vi "获取MPPT状态.vi"(8 "error in (no error)":errorcluster, 11 "MB session in":refnum<class "MB_Master.lvclass">) -> (0 "error out":errorcluster, 1 "结果字符串":string caption="状态", 2 "状态":T1, 3 "MB session out":refnum<class "MB_Master.lvclass">)   [LabVIEW 2016, in "采配水.lvlib"]
uses:
  <vilib>/Plasmionique/MB Master/MB_Master/MB_Master.lvclass
  <vilib>/Plasmionique/MB Master/MB Master.lvlib
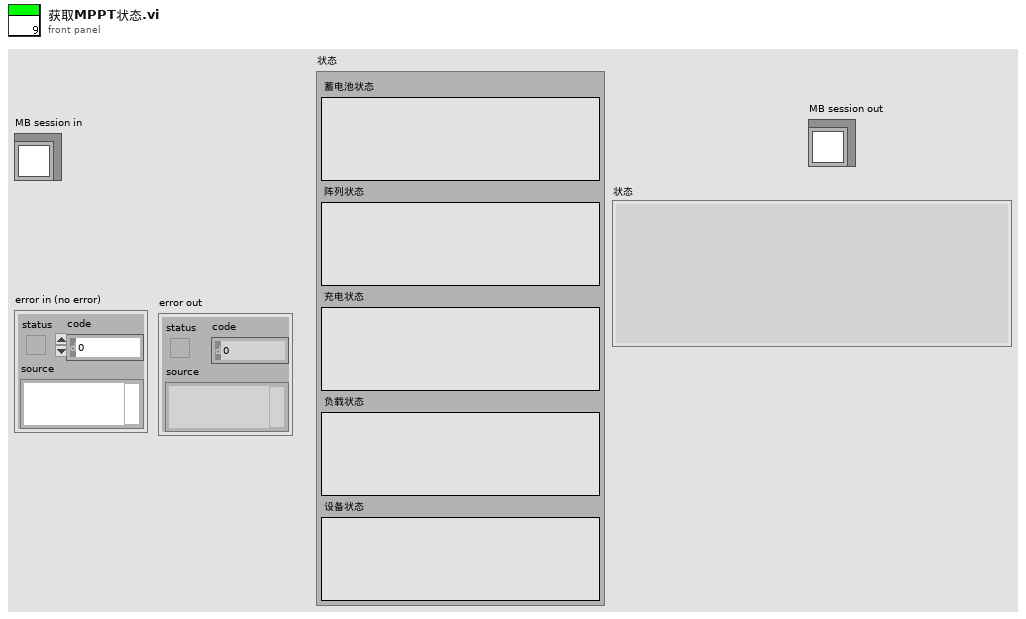
[diagram p1: front panel]
types:
  T1 = cluster{"蓄电池状态":string, "阵列状态":string, "充电状态":string, "负载状态":string, "设备状态":string}
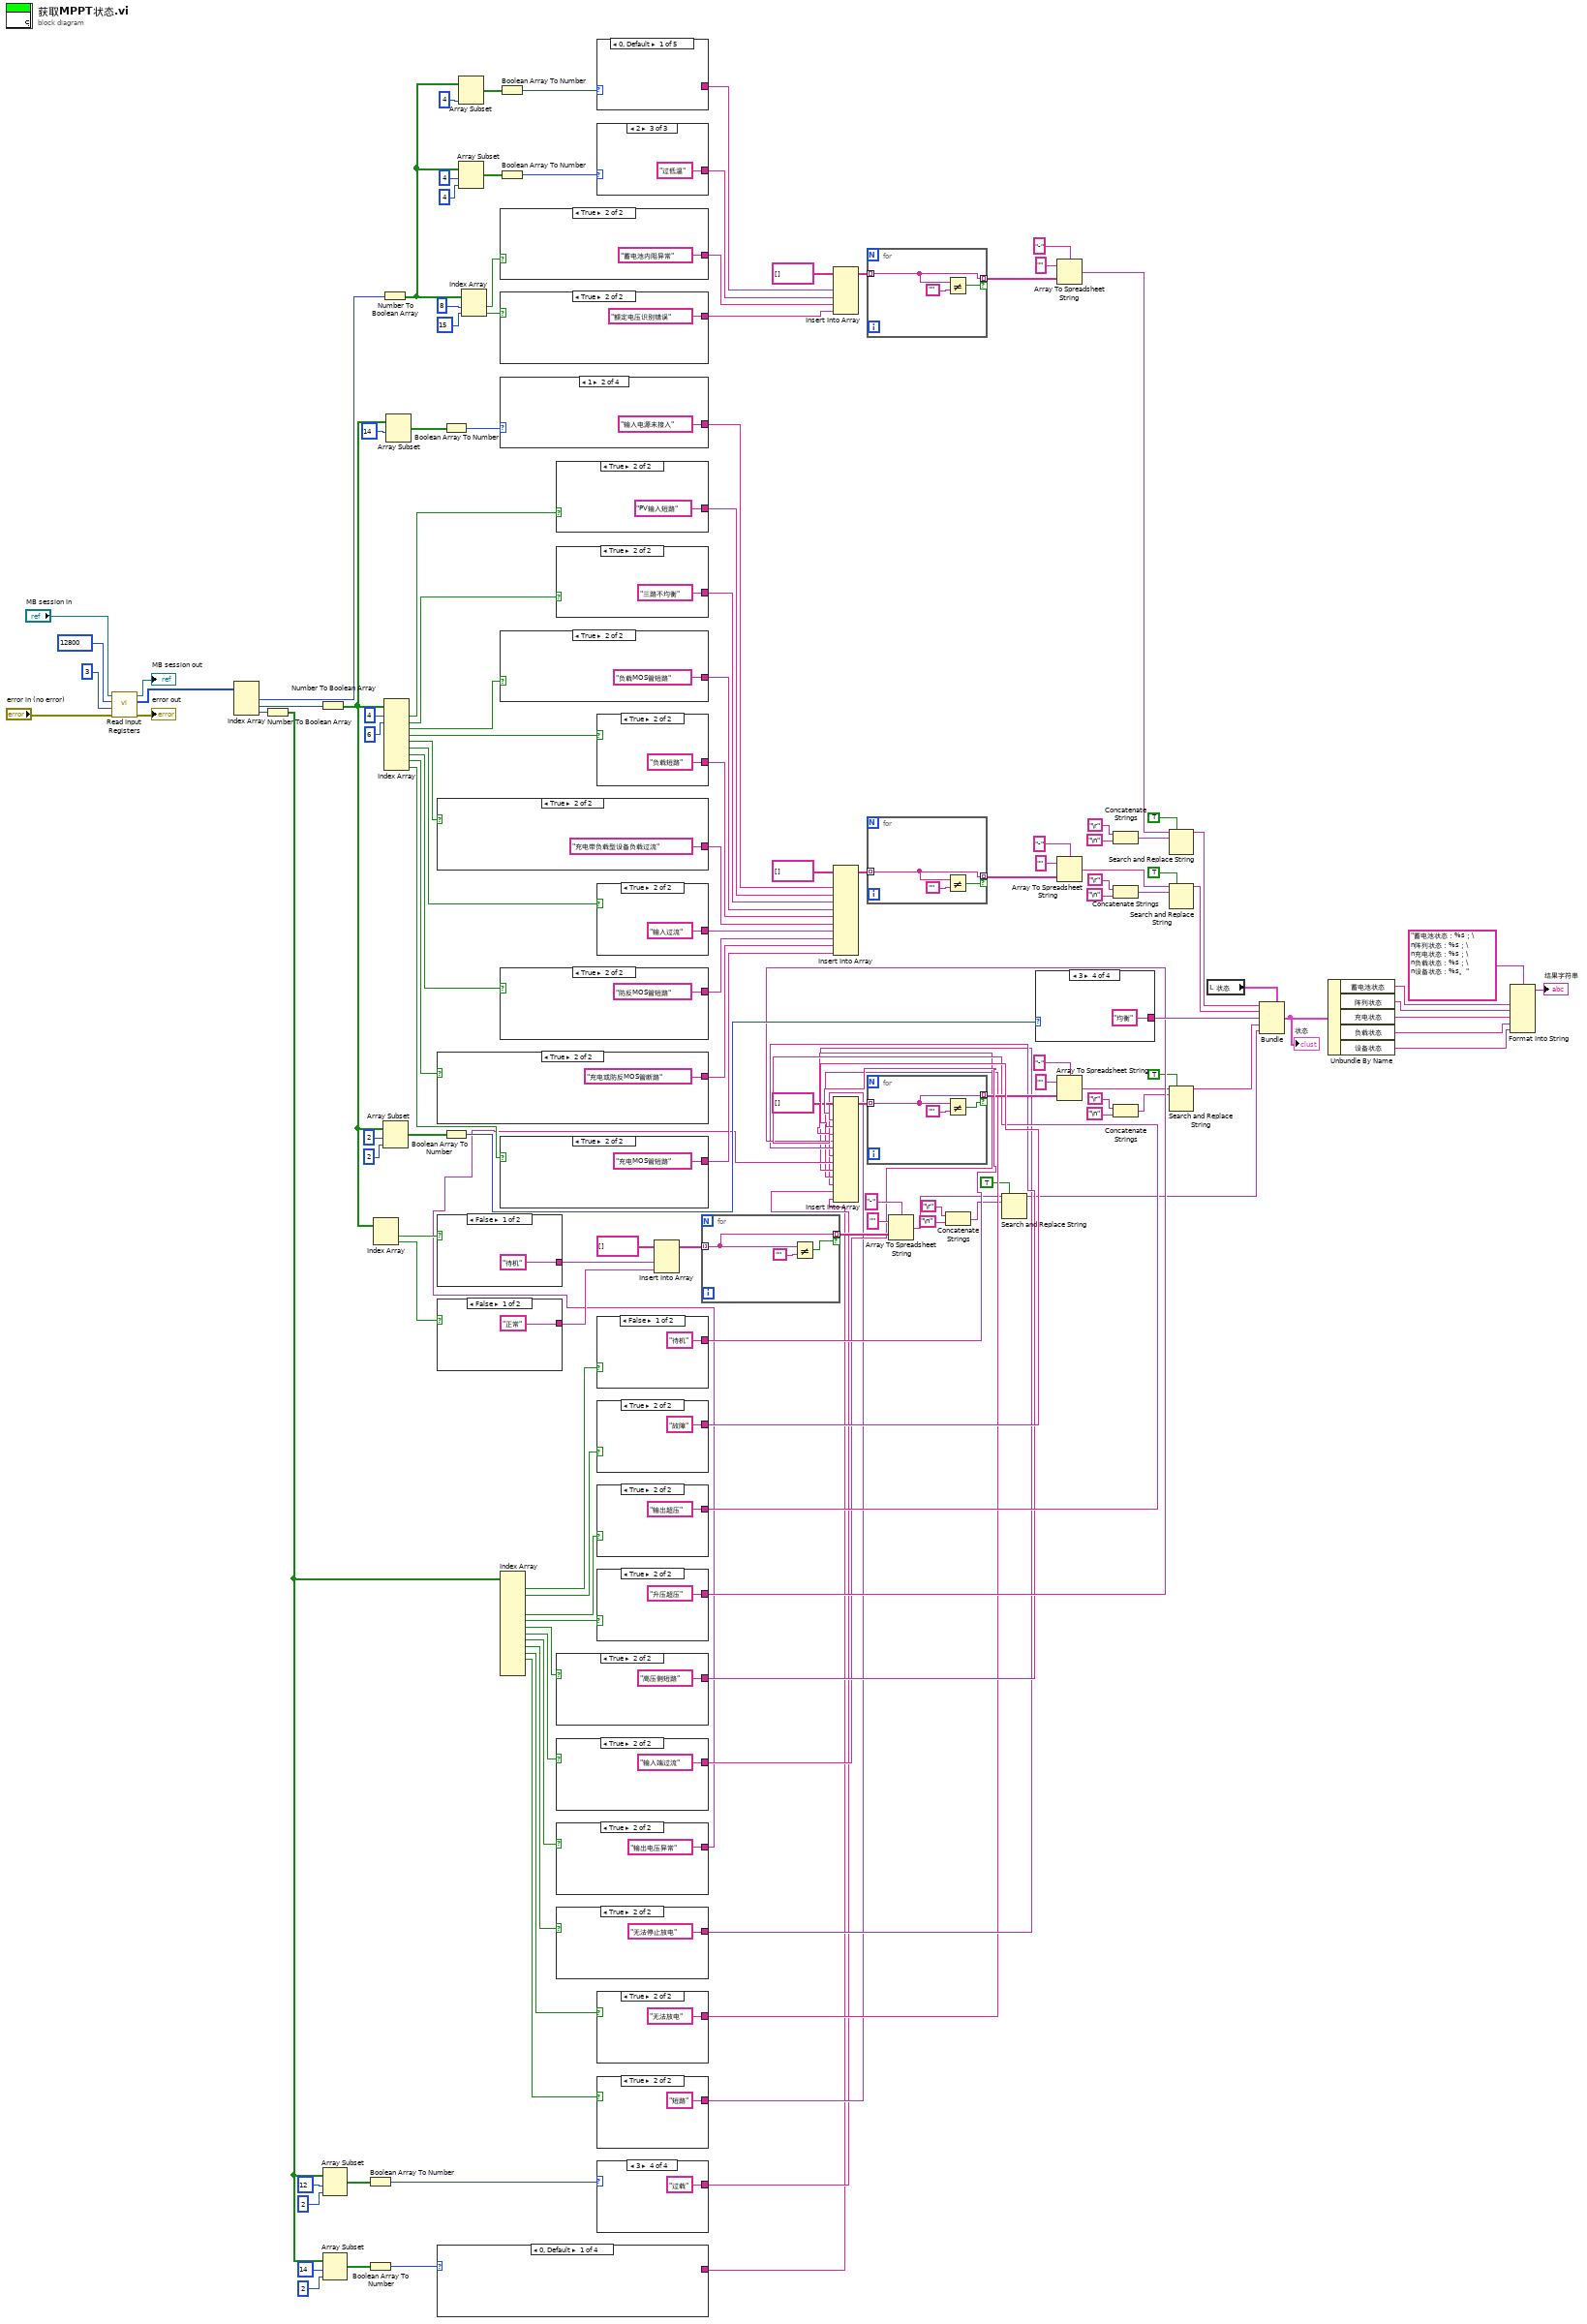
[diagram p0: block diagram]
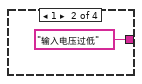
[diagram p2: hidden frame]
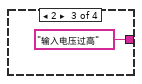
[diagram p3: hidden frame]
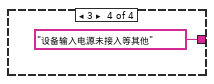
[diagram p4: hidden frame]
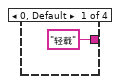
[diagram p5: hidden frame]
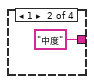
[diagram p6: hidden frame]
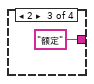
[diagram p7: hidden frame]
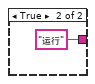
[diagram p17: hidden frame]
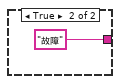
[diagram p18: hidden frame]
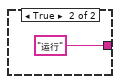
[diagram p19: hidden frame]
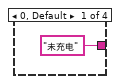
[diagram p20: hidden frame]
diagram:
  n1 = call <vilib>:"Read Input Registers.vi"("error in (no error)"="error in (no error)", "quantity"=u16 3, "starting address"=u16 12800, "MB session in"="MB session in") -> ("error out"=→"error out":errorcluster, "Registers"=w138:u16[], "MB session out"=→"MB session out":refnum<class "MB_Master.lvclass">)  [unwired: 5 in]
  n2 = Index Array(array=w138) -> (element #1=w137:u16, element #2=w115:u16, element #3=w70:u16)  [unwired: 3 in]
  n3 = Number To Boolean Array(number=w70) -> (Boolean array=w44:bool[])
  n4 = Number To Boolean Array(number=w115) -> (Boolean array=w81:bool[])
  n5 = Array Subset(array=w44, index=12 ("索引"), length=2 ("长度")) -> (w50:bool[])
  n6 = Array Subset(array=w44, index=14 ("索引"), length=2 ("长度")) -> (w47:bool[])
  n7 = Boolean Array To Number(Boolean array=w50) -> (number=w49:u32)
  n8 = Boolean Array To Number(Boolean array=w47) -> (number=w48:u32)
  n9 = Index Array(array=w81) -> (element #1=w80:bool, element #2=w79:bool)  [unwired: 2 in]
  n10 = Number To Boolean Array(number=w137) -> (Boolean array=w130:bool[])
  n11 = Array Subset(array=w81, index=2 ("索引"), length=2 ("长度")) -> (w84:bool[])
  n12 = Index Array(array=w81, index #1=4 ("索引"), index #2=6 ("索引")) -> (element #1=w101:bool, element #2=w110:bool, element #3=w109:bool, element #4=w108:bool, element #5=w107:bool, element #6=w106:bool, element #7=w105:bool, element #8=w104:bool, element #9=w103:bool)  [unwired: 7 in]
  n13 = Array Subset(array=w81, index=14 ("索引")) -> (w113:bool[])  [unwired: 1 in]
  n14 = case shown="True" w107 {
    tunnel: [_ "充电带负载型设备负载过流"] -> w91
    frame False {
    }
    frame True {
    }
  }
  n15 = case shown="True" w104 {
    tunnel: [_ "充电或防反MOS管断路"] -> w88
    frame False {
    }
    frame True {
    }
  }
  n16 = case shown="False" w80 {
    tunnel: ["待机" "运行"] -> w72
    frame False {
    }
    frame True {
    }
  }
  n17 = case shown="False" w79 {
    tunnel: ["正常" "故障"] -> w71
    frame False {
    }
    frame True {
    }
  }
  n18 = case shown="0, Default" w48 {
    tunnel: [_ "输入电压过低" "输入电压过高" "设备输入电源未接入等其他"] -> w34
    frame 0, Default {
    }
    frame 1 {
    }
    frame 2 {
    }
    frame 3 {
    }
  }
  n19 = Boolean Array To Number(Boolean array=w113) -> (number=w112:u32)
  n20 = Boolean Array To Number(Boolean array=w84) -> (number=w83:u32)
  n21 = Array Subset(array=w130, length=4 ("长度")) -> (w135:bool[])  [unwired: 1 in]
  n22 = Array Subset(array=w130, index=4 ("长度"), length=4 ("长度")) -> (w131:bool[])
  n23 = Index Array(array=w130, index #1=8 ("索引"), index #2=15 ("索引")) -> (element #1=w129:bool, element #2=w126:bool)
  n24 = Boolean Array To Number(Boolean array=w135) -> (number=w134:u32)
  n25 = Boolean Array To Number(Boolean array=w131) -> (number=w116:u32)
  n26 = case shown="True" w129 {
    tunnel: [_ "蓄电池内阻异常"] -> w122
    frame False {
    }
    frame True {
    }
  }
  n27 = case shown="True" w126 {
    tunnel: [_ "额定电压识别错误"] -> w121
    frame False {
    }
    frame True {
    }
  }
  n28 = case shown="1" w112 {
    tunnel: [_ "输入电源未接入" "输入电压过高" "输入电压错误"] -> w78
    frame 0, Default {
    }
    frame 1 {
    }
    frame 2 {
    }
    frame 3 {
    }
  }
  n29 = case shown="True" w109 {
    tunnel: [_ "负载MOS管短路"] -> w93
    frame False {
    }
    frame True {
    }
  }
  n30 = case shown="True" w105 {
    tunnel: [_ "防反MOS管短路"] -> w89
    frame False {
    }
    frame True {
    }
  }
  n31 = case shown="True" w103 {
    tunnel: [_ "充电MOS管短路"] -> w87
    frame False {
    }
    frame True {
    }
  }
  n32 = Index Array(array=w44) -> (element #1=w61:bool, element #2=w62:bool, element #5=w60:bool, element #6=w59:bool, element #7=w58:bool, element #8=w57:bool, element #9=w56:bool, element #10=w55:bool, element #11=w54:bool, element #12=w53:bool)  [unwired: 14 in, 4 out]
  n33 = case shown="True" w101 {
    tunnel: [_ "PV输入短路"] -> w95
    frame False {
    }
    frame True {
    }
  }
  n34 = case shown="True" w110 {
    tunnel: [_ "三路不均衡"] -> w94
    frame False {
    }
    frame True {
    }
  }
  n35 = case shown="True" w58 {
    tunnel: [_ "高压侧短路"] -> w41
    frame False {
    }
    frame True {
    }
  }
  n36 = case shown="True" w57 {
    tunnel: [_ "输入端过流"] -> w40
    frame False {
    }
    frame True {
    }
  }
  n37 = case shown="True" w56 {
    tunnel: [_ "输出电压异常"] -> w39
    frame False {
    }
    frame True {
    }
  }
  n38 = case shown="True" w55 {
    tunnel: [_ "无法停止放电"] -> w38
    frame False {
    }
    frame True {
    }
  }
  n39 = case shown="0, Default" w134 {
    tunnel: [_ "超压" "欠压" "过放" "错误"] -> w125
    frame 0, Default {
    }
    frame 1 {
    }
    frame 2 {
    }
    frame 3 {
    }
    frame 4 {
    }
  }
  n40 = case shown="2" w116 {
    tunnel: [_ "过高温" "过低温"] -> w123
    frame 0, Default {
    }
    frame 1 {
    }
    frame 2 {
    }
  }
  n41 = case shown="True" w108 {
    tunnel: [_ "负载短路"] -> w92
    frame False {
    }
    frame True {
    }
  }
  n42 = case shown="True" w106 {
    tunnel: [_ "输入过流"] -> w90
    frame False {
    }
    frame True {
    }
  }
  n43 = case shown="False" w61 {
    tunnel: ["待机" "运行"] -> w68
    frame False {
    }
    frame True {
    }
  }
  n44 = case shown="True" w62 {
    tunnel: [_ "故障"] -> w69
    frame False {
    }
    frame True {
    }
  }
  n45 = case shown="True" w60 {
    tunnel: [_ "输出超压"] -> w43
    frame False {
    }
    frame True {
    }
  }
  n46 = case shown="True" w59 {
    tunnel: [_ "升压超压"] -> w42
    frame False {
    }
    frame True {
    }
  }
  n47 = case shown="True" w54 {
    tunnel: [_ "无法放电"] -> w37
    frame False {
    }
    frame True {
    }
  }
  n48 = case shown="True" w53 {
    tunnel: [_ "短路"] -> w36
    frame False {
    }
    frame True {
    }
  }
  n49 = case shown="3" w49 {
    tunnel: ["轻载" "中度" "额定" "过载"] -> w35
    frame 0, Default {
    }
    frame 1 {
    }
    frame 2 {
    }
    frame 3 {
    }
  }
  n50 = Insert Into Array(array=string[] [] ("数组"), new element #1=w72, new element #2=w71) -> (w74:string[])  [unwired: 1 in]
  n51 = for {
    tunnel: w74 -> [w188] mode=indexing
    tunnel: [w188] -> w75 mode=indexing if=w187
    n52 = Not Equal?(x=w188, y="") -> (x != y?=w187:bool)
  }
  n53 = Insert Into Array(array=string[] [] ("数组"), new element #1=w125, new element #2=w123, new element #3=w122, new element #4=w121) -> (w120:string[])  [unwired: 1 in]
  n54 = Insert Into Array(array=string[] [] ("数组"), new element #1=w78, new element #2=w95, new element #3=w94, new element #4=w93, new element #5=w92, new element #6=w91, new element #7=w90, new element #8=w89, new element #9=w88, new element #10=w87) -> (w99:string[])  [unwired: 1 in]
  n55 = Insert Into Array(array=string[] [] ("数组"), new element #1=w68, new element #2=w69, new element #3=w43, new element #4=w42, new element #5=w41, new element #6=w40, new element #7=w39, new element #8=w38, new element #9=w37, new element #10=w36, new element #11=w35, new element #12=w34) -> (w66:string[])  [unwired: 1 in]
  n56 = for {
    tunnel: w120 -> [w191] mode=indexing
    tunnel: [w191] -> w119 mode=indexing if=w190
    n57 = Not Equal?(x=w191, y="") -> (x != y?=w190:bool)
  }
  n58 = for {
    tunnel: w99 -> [w194] mode=indexing
    tunnel: [w194] -> w98 mode=indexing if=w193
    n59 = Not Equal?(x=w194, y="") -> (x != y?=w193:bool)
  }
  n60 = for {
    tunnel: w66 -> [w197] mode=indexing
    tunnel: [w197] -> w65 mode=indexing if=w196
    n61 = Not Equal?(x=w197, y="") -> (x != y?=w196:bool)
  }
  n62 = Array To Spreadsheet String(delimiter (Tab)="-" ("分隔符(Tab)"), array=w75, 3:"" ("格式字符串")) -> (spreadsheet string=w14:string)
  n63 = Concatenate Strings("\r", "\n") -> (w19:string)
  n64 = Search and Replace String(replace all?=TRUE ("替换全部？(F)"), input string=w14, search string=w19) -> (result string=w13:string)  [unwired: 5 in, 3 out]
  n65 = case shown="3" w83 {
    tunnel: ["未充电" "浮充" "提升" "均衡"] -> w82
    frame 0, Default {
    }
    frame 1 {
    }
    frame 2 {
    }
    frame 3 {
    }
  }
  n66 = Array To Spreadsheet String(delimiter (Tab)="-" ("分隔符(Tab)"), array=w119, 3:"" ("格式字符串")) -> (spreadsheet string=w8:string)
  n67 = Array To Spreadsheet String(delimiter (Tab)="-" ("分隔符(Tab)"), array=w98, 3:"" ("格式字符串")) -> (spreadsheet string=w2:string)
  n68 = Array To Spreadsheet String(delimiter (Tab)="-" ("分隔符(Tab)"), array=w65, 3:"" ("格式字符串")) -> (spreadsheet string=w24:string)
  n69 = Concatenate Strings("\r", "\n") -> (w9:string)
  n70 = Concatenate Strings("\r", "\n") -> (w6:string)
  n71 = Concatenate Strings("\r", "\n") -> (w20:string)
  n72 = Search and Replace String(replace all?=TRUE ("替换全部？(F)"), input string=w8, search string=w9) -> (result string=w7:string)  [unwired: 5 in, 3 out]
  n73 = Search and Replace String(replace all?=TRUE ("替换全部？(F)"), input string=w2, search string=w6) -> (result string=w1:string)  [unwired: 5 in, 3 out]
  n74 = Search and Replace String(replace all?=TRUE ("替换全部？(F)"), input string=w24, search string=w20) -> (result string=w15:string)  [unwired: 5 in, 3 out]
  n75 = local read "状态"() -> (w32:T1)
  n76 = Bundle(cluster=w32, "蓄电池状态"=w7, "阵列状态"=w1, "充电状态"=w82, "负载状态"=w15, "设备状态"=w13) -> (w31:T1)
  "状态" <- w31
  n77 = Unbundle By Name(w31) -> ("蓄电池状态"=w30:string, "阵列状态"=w29:string, "充电状态"=w28:string, "负载状态"=w27:string, "设备状态"=w26:string)
  n78 = Format Into String(format string="蓄电池状态：%s；\n阵列状态：%s；\n充电状态：%s；\n负载状态：%s；\n设备状态：%s。" ("格式字符串"), w30, w29, w28, w27, w26) -> (resulting string=→"结果字符串":string)  [unwired: 2 in, 1 out]
